vi "LabVIEW Real-Time Serial Close.vi"(8 "error out":errorcluster, 11 "FPGA Main Ref":T1) -> (0 "error out":errorcluster)   [LabVIEW 2012]
doc: "Close connection to the serial port."
uses:
  Program Files (x86)/National Instruments/LabVIEW 2012/examples/robotics/RS-232 with DIO/FPGA Main VI Reference Typedef.ctl
  <vilib>/Utility/error.llb/Error Cluster From Error Code.vi
  <vilib>/rvi/errors/niLvFpgaAdjustHostInterfaceError.vi
  <vilib>/FPGAPlugInAG/sbRIO-9631/niLvFpga_Close_sbRIO-9631.vi
  <vilib>/rvi/interface/nirviReadWriteControl/nirviReadWriteControl.xnode
  Program Files (x86)/National Instruments/LabVIEW 2012/examples/robotics/RS-232 with DIO/FPGA Bitfiles/FPGARS232_FPGATarget_RS-232FPGAMain_GZpp3UKya7w.lvbitx
  Program Files (x86)/National Instruments/LabVIEW 2012/examples/robotics/RS-232 with DIO/RS-232 FPGA Main.vi
  <vilib>/rvi/interface/nirviCloseFPGA/nirviCloseFPGA.xnode
  NiFpgaLv.dll
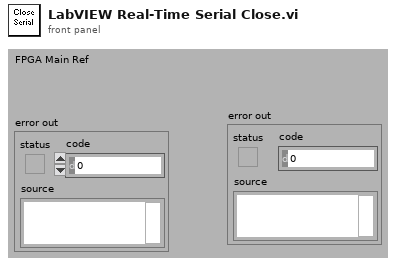
[diagram p1: front panel]
types:
  T1 = typedef "FPGA Main VI Reference Typedef.ctl" = refnum<k20>
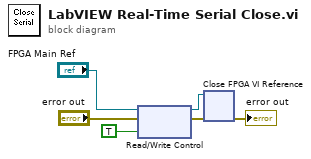
[diagram p0: block diagram]
diagram:
  n1 = xnode "Read/Write Control"("FPGA VI Reference In"="FPGA Main Ref", "error in"="error out", "stop"=TRUE) -> ("FPGA VI Reference Out"=w4:T1, "error out"=w5:errorcluster)
  n2 = xnode "Close FPGA VI Reference"("FPGA VI Reference In"=w4, "error in"=w5) -> ("error out"=→"error out":errorcluster)
